vi "inliner.vi"() -> ()   [LabVIEW 2013]
panel:
  out "error out":errorcluster
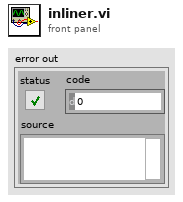
[diagram p1: front panel]
types:
  T1 = enum16{"Share clones between instances", "Preallocate clone for each instance"}
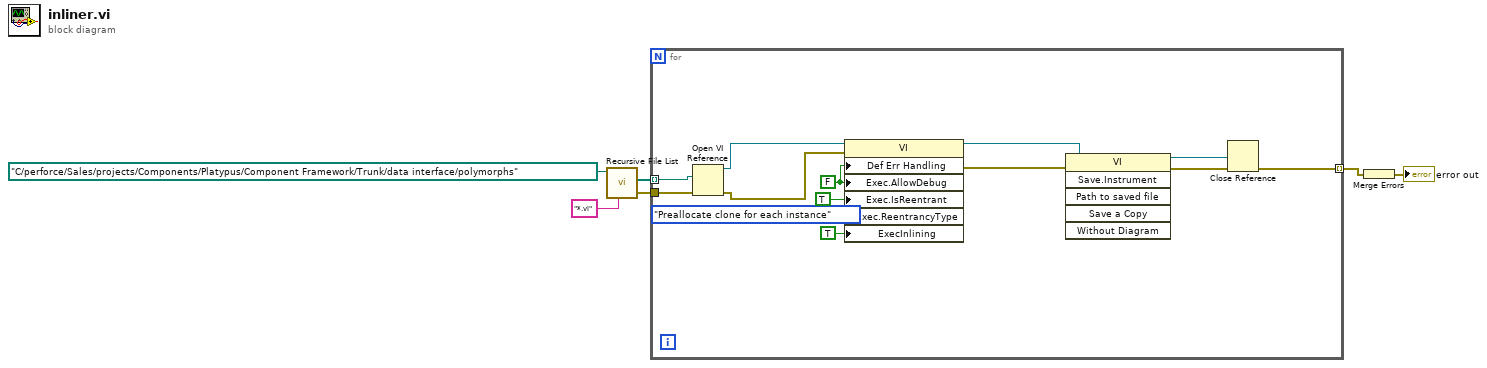
[diagram p0: block diagram]
diagram:
  n1 = call <vilib>:"Recursive File List.vi"("pattern"="*.vi", "Folder Path"=path "C:/perforce/Sales/projects/Components/Platypus/Component Framework/Trunk/data interface/polymorphs") -> ("error out"=w3:errorcluster, "All Files in Dir"=w4:path[])  [unwired: 5 in, 3 out]
  n2 = for {
    tunnel: w4 -> [w19] mode=indexing
    tunnel: w3 -> [w18]
    tunnel: [w8] -> w2 mode=indexing
    w7 = FALSE ("Execution:Allow Debugging")
    n3 = Open VI Reference(vi path=w19, error in (no error)=w18) -> (vi reference=w17:refnum<vi>, error out=w16:errorcluster)  [unwired: 4 in]
    n4 = property class="VI"(reference=w17, error in=w16, "Def Err Handling"=w7, "Exec.AllowDebug"=w7, "Exec.IsReentrant"=TRUE ("Execution:Is Reentrant"), "Exec.ReentrancyType"=T1."Preallocate clone for each instance" ("Execution:Reentrancy Type"), "ExecInlining"=TRUE ("Execution:Inline SubVI")) -> (reference out=w12:refnum<vi>, error out=w11:errorcluster)
    n5 = invoke class="VI" method="Save.Instrument"(reference=w12, error in=w11) -> (reference out=w10:refnum<vi>, error out=w9:errorcluster)  [unwired: 4 in, 4 out]
    n6 = Close Reference(reference=w10, error in (no error)=w9) -> (error out=w8:errorcluster)
  }
  n7 = Merge Errors(w2) -> (→"error out":errorcluster)
